vi "TW Generate proto file.vi"(8 "error in":errorcluster, 10 "New Subname":string, 11 "Template Project Path":path) -> (0 "error out":errorcluster, 2 "gRPC Service Name":string, 3 "proto File Path":path)   [LabVIEW 2021, in "Plugin Generator.lvlib"]
uses:
  Plugin Generator.lvlib
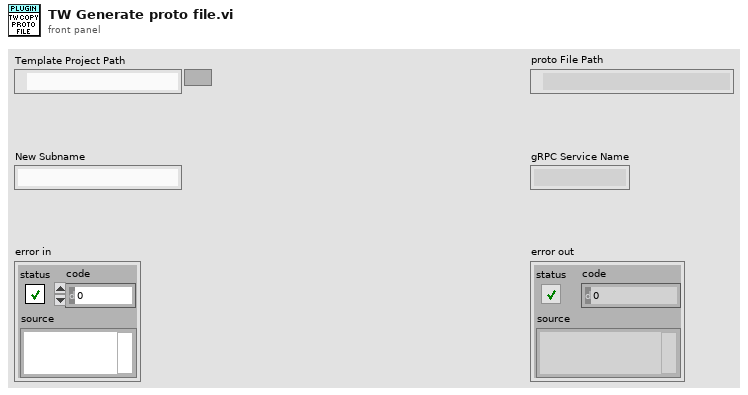
[diagram p1: front panel]
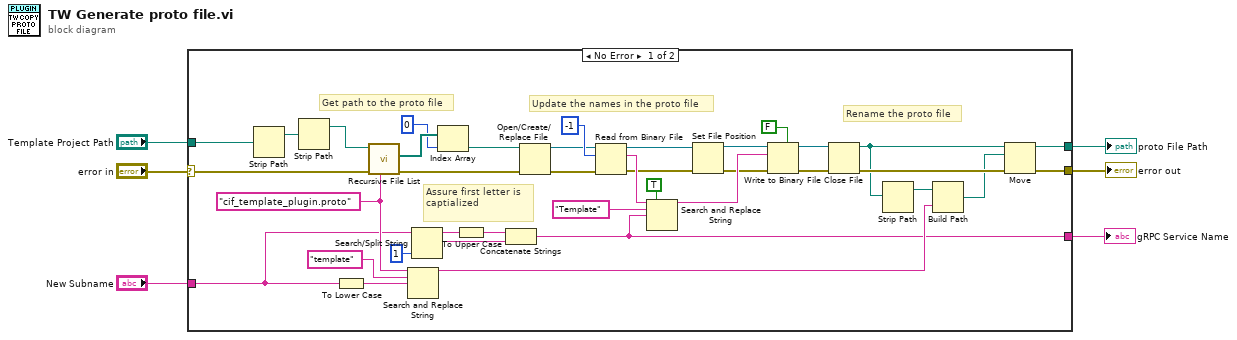
[diagram p0: block diagram]
diagram:
  n1 = case shown="No Error" "error in" {
    selector: "error in" -> [w9 w45]
    tunnel: [w16 w45] -> w6
    tunnel: [w15 _] -> w5
    tunnel: "New Subname" -> [w24 _]
    tunnel: "Template Project Path" -> [w8 _]
    tunnel: [w7 _] -> w1
    frame No Error {
      w35 = "cif_template_plugin.proto" ("pattern")
      # "Rename the proto file"
      # "Update the names in the proto file"
      # "Get path to the proto file"
      # "Assure first letter is captialized"
      n2 = Strip Path(path=w8) -> (stripped path=w27:path)  [unwired: 1 out]
      n3 = Strip Path(path=w27) -> (stripped path=w26:path)  [unwired: 1 out]
      n4 = To Lower Case(string=w24) -> (all lower case string=w32:string)
      n5 = call <vilib>:"Recursive File List.vi"("pattern"=w35, "error in (no error)"=w9, "Folder Path"=w26) -> ("error out"=w14:errorcluster, "All Files in Dir"=w44:path[])  [unwired: 4 in, 3 out]
      n6 = Search and Replace String(input string=w35, search string="template", replace string=w32) -> (result string=w33:string)  [unwired: 5 in, 3 out]
      n7 = Search/Split String(string=w24, offset (0)=1 ("length (rest)")) -> (substring before match=w30:string, match + rest of string=w28:string)  [unwired: 1 in, 1 out]
      n8 = Index Array(array=w44, index=0) -> (element=w10:path)
      n9 = To Upper Case(1:w30) -> (0:w29:string)
      n10 = Concatenate Strings(w29, w28) -> (w7:string)
      n11 = Open/Create/Replace File(file path (use dialog)=w10, error in=w14) -> (refnum out=w11:refnum<file>, error out=w13:errorcluster)  [unwired: 4 in, 1 out]
      n12 = Read from Binary File(8:w13, 10:-1 ("count (1)"), 11:w11) -> (0:w22:errorcluster, 2:w42:string, 3:w23:refnum<file>)  [unwired: 3 in, 1 out]
      n13 = Search and Replace String(replace all?=TRUE ("replace all? (F)"), input string=w42, search string="Template", replace string=w7) -> (result string=w38:string)  [unwired: 4 in, 3 out]
      n14 = Set File Position(refnum=w23, error in=w22) -> (refnum out=w21:refnum<file>, error out=w20:errorcluster)  [unwired: 2 in]
      n15 = Write to Binary File(file (use dialog)=w21, data=w38, error in=w20, 5:FALSE ("prepend array or string size? (T)")) -> (refnum out=w40:refnum<file>, error out=w39:errorcluster)  [unwired: 2 in, 1 out]
      n16 = Close File(refnum=w40, error in=w39) -> (path=w18:path, error out=w19:errorcluster)
      n17 = Strip Path(path=w18) -> (stripped path=w25:path)  [unwired: 1 out]
      n18 = Build Path(base path=w25, name or relative path=w33) -> (appended path=w17:path)
      n19 = Move(source path=w18, error in=w19, 10:w17) -> (error out=w16:errorcluster, 3:w15:path)  [unwired: 2 in, 1 out]
    }
    frame Error {
    }
  }
  "error out" <- w6
  "proto File Path" <- w5
  "gRPC Service Name" <- w1
